vi "Control_ArduinoRobot_by_DS4.vi"() -> ()   [LabVIEW 2019]
uses:
  <vilib>/MakerHub/LINX/Public/Peripherals/Digital/Digital Write 1 Chan.vi
  <vilib>/MakerHub/LINX/Public/Peripherals/Digital/Digital Write N Chans.vi
  <vilib>/MakerHub/LINX/Private/Local IO/LinxDigitalWrite.vi
  <vilib>/MakerHub/LINX/Public/Utilities/Check Channel.vi
  <vilib>/MakerHub/LINX/Public/Utilities/Open Serial.vi
  <vilib>/MakerHub/PS4-Controller/Public/Open First Controller.vi
  <vilib>/MakerHub/LINX/Private/Utilties/Generate Error.vi
  <vilib>/MakerHub/PS4-Controller/LMH-PS4.lvlib
  <vilib>/MakerHub/LINX/LMH-LINX.lvlib
panel:
  out "Buzz":bool
  out "Laser":bool
  out "Right":bool
  out "Left":bool
  out "Backward":bool
  out "Forward":bool
  in  "stop":bool
  in  "Serial Port":refnum<visa-resource-name>="N/A"
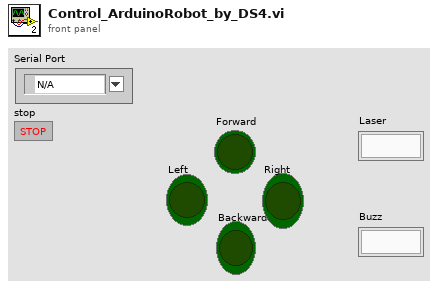
[diagram p1: front panel]
types:
  T1 = typedef "LMH-LINX.lvlib/LINX Ref.ctl" = cluster{"IO":T2, "Interface":T3, "LINX Device Config":T4}
  T2 = typedef "LMH-LINX.lvlib/Platform.ctl" = enum16{"Remote", "Local"}
  T3 = typedef "LMH-LINX.lvlib/Interface.ctl" = enum16{"Serial", "TCP"}
  T4 = typedef "LMH-LINX.lvlib/Device.lvlib/LINX Device Config.ctl" = cluster{"Interface":T3, "COM Port":refnum<visa-resource-name>, "TCP Configuration":T5, "Device Family":u8, "Device ID":u8, "Device Name":string, "TCP Ref":refnum<k5>, "Channels":T6}
  T5 = typedef "LMH-LINX.lvlib/Device.lvlib/TCP Config.ctl" = cluster{"IP Address":string, "Port":u16}
  T6 = typedef "LMH-LINX.lvlib/Channels.ctl" = cluster{"DI":u8[], "DO":u8[], "AI":u8[], "AO":u8[], "PWM":u8[], "QE":u8[], "UART":u8[], "I2C 2":u8[], "SPI":u8[], "CAN":u8[], "Servo":u8[], "AI Ref (V)":dbl, "AI Resolution (Bits)":u8, "AO Ref (V)":dbl, "AO Resolution (Bits)":u8}
  T7 = typedef "LMH-PS4.lvlib/PS4 Controller Ref.ctl" = cluster{"Controller Ref":refnum<k1>, "PS4 Events Ref":refnum<event-registration>, "Worker Ref":refnum<vi>}
  T8 = typedef "LMH-PS4.lvlib/Buttons.ctl" = cluster{"Square":bool, "X":bool, "Circle":bool, "Triangle":bool, "L1":bool, "R1":bool, "L2":bool, "R2":bool, "Share":bool, "Options":bool, "Left Thumbstick":bool, "Right Thumbstick":bool, "Playstation Button":bool, "Pad":bool}
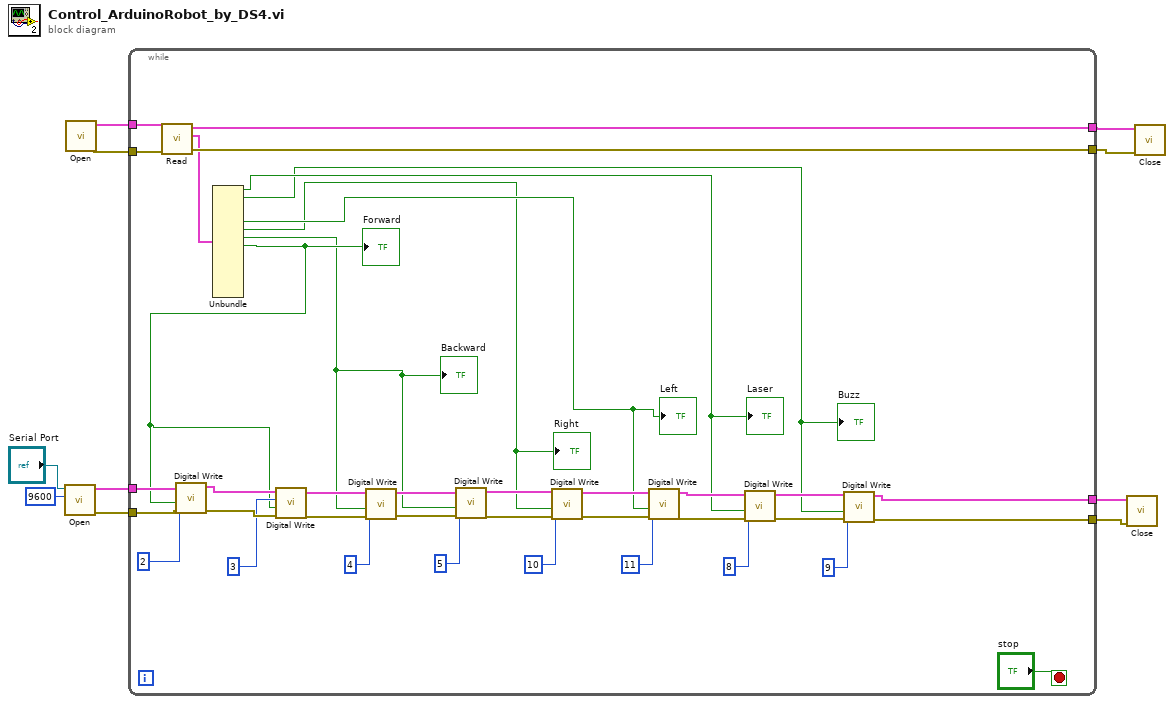
[diagram p0: block diagram]
diagram:
  n1 = call-poly <vilib>:"Open.vi"("Baud Rate Override"=u32 9600, "Serial Port"="Serial Port") -> ("Error Out"=w3:errorcluster, "LINX Resource"=w4:T1)  [unwired: 7 in, 1 out]
  n2 = call-poly <vilib>:"Open.vi"() -> ("Error Out"=w9:errorcluster, "PS4 Controller Ref"=w10:T7)  [unwired: 9 in, 1 out]
  n3 = while {
    tunnel: w10 -> [w48]
    tunnel: w9 -> [w47]
    tunnel: [w46] -> w8
    tunnel: [w45] -> w7
    tunnel: w4 -> [w43]
    tunnel: w3 -> [w42]
    tunnel: [w12] -> w2
    tunnel: [w11] -> w1
    stop <- "stop" stop-if-true
    n4 = call <vilib>:"Read.vi"("Error In"=w47, "PS4 Controller Ref"=w48) -> ("Error Out"=w45:errorcluster, "Buttons"=w44:T8, "PS4 Controller Ref"=w46:T7)  [unwired: 6 in, 1 out]
    n5 = Unbundle(w44) -> ("Square"=w14:bool, "X"=w13:bool, "L1"=w22:bool, "R1"=w21:bool, "L2"=w29:bool, "R2"=w36:bool)  [unwired: 8 out]
    "Forward" <- w36
    "Backward" <- w29
    "Left" <- w22
    "Right" <- w21
    "Laser" <- w14
    "Buzz" <- w13
    n6 = call-poly <vilib>:"Digital Write.vi"("Error In"=w42, "Output Value"=w36, "DO Channel"=u8 2, "LINX Resource"=w43) -> ("Error Out"=w40:errorcluster, "LINX Resource"=w41:T1)  [unwired: 6 in]
    n7 = call-poly <vilib>:"Digital Write.vi"("Error In"=w40, "Output Value"=w36, "DO Channel"=u8 3, "LINX Resource"=w41) -> ("Error Out"=w32:errorcluster, "LINX Resource"=w35:T1)  [unwired: 6 in]
    n8 = call-poly <vilib>:"Digital Write.vi"("Error In"=w32, "Output Value"=w29, "DO Channel"=u8 4, "LINX Resource"=w35) -> ("Error Out"=w33:errorcluster, "LINX Resource"=w34:T1)  [unwired: 6 in]
    n9 = call-poly <vilib>:"Digital Write.vi"("Error In"=w33, "Output Value"=w29, "DO Channel"=u8 5, "LINX Resource"=w34) -> ("Error Out"=w25:errorcluster, "LINX Resource"=w28:T1)  [unwired: 6 in]
    n10 = call-poly <vilib>:"Digital Write.vi"("Error In"=w25, "Output Value"=w21, "DO Channel"=u8 10, "LINX Resource"=w28) -> ("Error Out"=w26:errorcluster, "LINX Resource"=w27:T1)  [unwired: 6 in]
    n11 = call-poly <vilib>:"Digital Write.vi"("Error In"=w26, "Output Value"=w22, "DO Channel"=u8 11, "LINX Resource"=w27) -> ("Error Out"=w19:errorcluster, "LINX Resource"=w20:T1)  [unwired: 6 in]
    n12 = call-poly <vilib>:"Digital Write.vi"("Error In"=w19, "Output Value"=w14, "DO Channel"=u8 8, "LINX Resource"=w20) -> ("Error Out"=w16:errorcluster, "LINX Resource"=w17:T1)  [unwired: 6 in]
    n13 = call-poly <vilib>:"Digital Write.vi"("Error In"=w16, "Output Value"=w13, "DO Channel"=u8 9, "LINX Resource"=w17) -> ("Error Out"=w11:errorcluster, "LINX Resource"=w12:T1)  [unwired: 6 in]
  }
  n14 = call <vilib>:"Close.vi"("Error In"=w1, "LINX Resource"=w2) -> ()  [unwired: 9 in, 1 out]
  n15 = call <vilib>:"Close.vi"("Error In"=w7, "PS4 Controller Ref"=w8) -> ()  [unwired: 9 in, 1 out]
